vi "Result_Test.vi"(8 "error in (no error)":errorcluster caption="entrée d'erreur (pas d'erreur)", 11 "Generate_SN en entrée":refnum<class "Find_SN_In_Database.lvclass">) -> (0 "error out":errorcluster caption="sortie d'erreur", 3 "Generate_SN en sortie":refnum<class "Find_SN_In_Database.lvclass">)   [LabVIEW 2020, in "Library Test.lvlib" / "Find_SN_In_Database.lvclass"]
uses:
  Find_SN_In_Database.lvclass
  Test_Without_Instr/Test_Without_Inst.lvclass
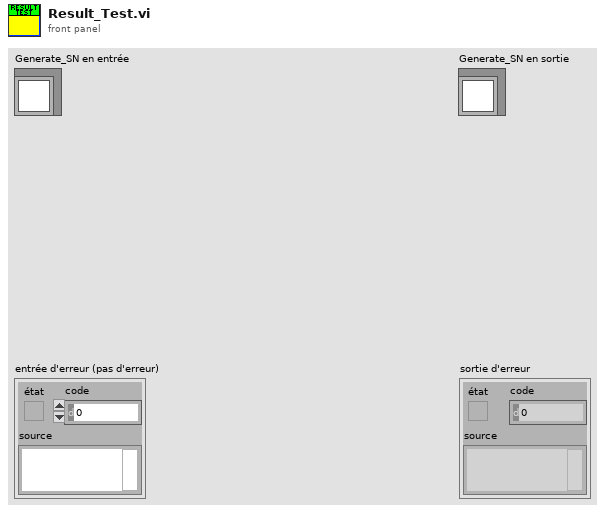
[diagram p1: front panel]
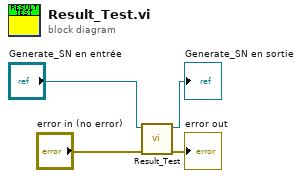
[diagram p0: block diagram]
diagram:
  n1 = call-parent "Result_Test.vi"("error in (no error)"="error in (no error)", "Test_Without_Inst en entrée"="Generate_SN en entrée") -> ("error out"=→"error out":errorcluster, "Test_Without_Inst en sortie"=→"Generate_SN en sortie":refnum<class "Find_SN_In_Database.lvclass">)  [unwired: 8 in]
